vi "CV.vi"(2 "Run uninterrupted?":bool, 3 "Device Category IN:":string(combo)="ATLAS18SS" caption="Device Category:", 4 "Batch No.:":string, 5 "Sensor Serial No.:":string, 6 "DB Serial No.:":string) -> (0 "Done!":bool)   [LabVIEW 2019]
doc: "Performs CV measurements according to ATLAS ITk Quality Control Specifications."
uses:
  general_VIs/globals/QC_MeasurementSetup.vi
  general_VIs/globals/QC_RunInformation.vi
  InstrControl/InstrumentSetup.vi
  InstrControl/Switching/Switching.lvclass
  InstrControl/SupplyControl/SupplyControl.lvclass
  InstrControl/LCRControl/LCRControl.lvclass
  InstrControl/ArduinoControl/ArduinoControl.lvclass
  <vilib>/Analysis/NI_AALBase.lvlib
  InstrControl/InstrControl.lvclass
panel:
  out "Tab Control 2":enum32{"CV Setup", "CV Scan"}(tab)
  in  "V_depletion limit [V]":dbl=-300.0
  in  "step interval [s] IN":i32=5 caption="step interval [s]"
  in  "step [V] IN":dbl=10.0 caption="step [V]" format="%.1f"
  in  "Final volts [V] IN":dbl=-500.0 caption="Final volts [V]"
  in  "Initial volts [V] IN":dbl caption="Initial volts [V]"
  in  "Current Limit [µA]":dbl=1000.0 min=0.0001 format="%.3f"
  in  "Continue":bool
  in  "Quit":bool
  in  "Software current limit?":bool
  in  "Frequency [Hz] Setup":i32=500 caption="Frequency [Hz]" format="%#.3p"
  in  "Measurement Configurations":bool
  out "RH":dbl[](array[numeric]) caption="RH [%]" format="%#.2f"
  out "step interval [s]":u32=5
  out "step [V]":dbl=10.0 format="%.1f"
  out "Final volts [V]":dbl=-700.0 format="%.1f"
  out "Initial volts [V]":dbl format="%.1f"
  out "Frequency [Hz]":i32=1000 format="%#.3p"
  out "Temp.":dbl[](array[numeric]) caption="Temp. [°C]" format="%#.2f"
  out "Volts":dbl[](array[numeric]) caption="Volts [V]"
  out "Resistance":dbl[](array[numeric]) caption="Res [kOhm]"
  out "Capacitance":dbl[](array[numeric]) caption="Cap [pF]"
  out "Cgraph":cluster{"Initial volts":dbl, dbl, dbl[]}(graph)
  in  "Scales":T1(ring)
  in  "Cscale":enum16{"1/C^2 [1/nF^2]", "nF", "pF"}(ring)
  out "positive ramp?":bool
  out "Tab Control":enum32{"CV Setup", "CV Scan"}(tab)
  in  "Switching":string(combo)="Pickering Matrix"
  in  "LCR Meter":string(combo)="WayneKerr 6440B"
  in  "User:":string(combo)="Christoph"
  in  "CV Supply":string(combo)="Keithley 2410"
  in  "Hardware Configurations":bool
  in  "Temperature":enum16{"Read Arduino", "Enter manually"}(ring)
  in  "Manufacturer:":string(combo)="Hamamatsu"
  in  "abort":bool
  out "Device Category:":string
  out "DB Serial No.:":string
  out "Current Volts:":dbl format="%.2f"
  in  "quit (no save)":bool
  in  "Quit & Save":bool
  out "Bias On/Off:":bool
  out "STATUS 1":string
  out "Initiated:":string
  out "Sensor No.:":string
  out "No of steps":u32
  out "Current reading No.":u32
  out "Last reading at:":string
  # "Strip Sensor QC: CV"
  # "University of\nCambridge"
  # "Vertical Scale:"
  # "Measurement Configuration"
  # "CV Scan parameters:"
  # "Last 5 readings:"
  # "n-4"
  # "n-3"
  # "n-2"
  # "n-1"
  # "n"
  # "DUT Description"
  # "Hardware"
  # "DUT & Test Description:"
  # "Current status:"
  # "Rdg No:"
  # "out of"
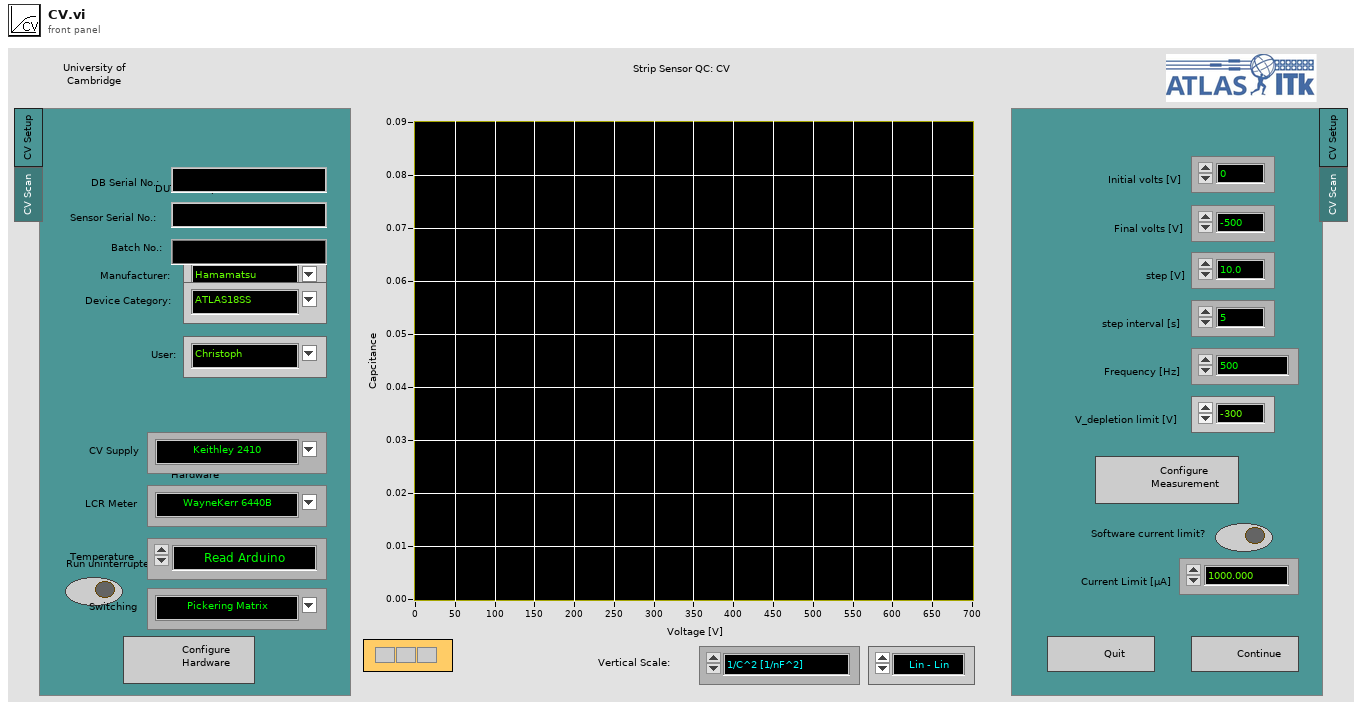
[diagram p1: front panel]
types:
  T1 = enum16{"Lin - Lin", "Log - Lin", "Lin - Log", "Log - log"}
  T2 = enum16{"Supply", "LCR", "Multimeter", "Switching"}
  T3 = enum16{"Reset", "Read Array", "Read Element", "Write Element", "Write Array", "Add Element", "Add Array"}
  T4 = enum16{"Reset", "Ground", "Striptest Bias", "Striptest SMU", "Striptest LCR", "IV", "CV", "Interstrip Cap", "Interstrip Res"}
  T5 = enum32{"IV", "CV", "Stability", "Striptest", "Cis", "Ris", "PTP"}
  T6 = cluster{"Sensor Serial No.:":string, "Wafer Serial No.:":string, "Batch:":string, "Manufacturer:":string, "Device Category:":string, "Database Serial No.:":string, "Date Initiated:":string, "Time Initiated:":string, "Test":string, "Instruments used:":string, "Probeplan used:":string, "End of Run comment:":string, "User:":string}
  T7 = cluster{"Institute":string, "Manufacturers":string[], "Devices":string[], "Serialnumbers Lookup DB":string, "Data directory":string, "Backup & screenshot directory":string, "List of known users":string[], "Measurement switch not used":bool, "Measurement Switch":string, "DUT Switch":string}
  T8 = cluster{"Supply":refnum<class "SupplyControl.lvclass">, "LCR":refnum<class "LCRControl.lvclass">, "Initial Voltage [V]":dbl, "Final Voltage [V]":dbl, "Step Size [V]":dbl, "Step Interval [s]":i32, "Number Of Steps":u32, "AC frequency [Hz]":i32, "RC Configuration":u16, "AC amplitude [V]":dbl, "Ramp down steps [V]":dbl, "Ramp down Interval [s]":i32, "Set Current Limit?":bool, "Current Limit [µA]":dbl, "Temperature Readout":enum16{"Read Arduino", "Enter manually"}, "Arduino":refnum<class "ArduinoControl.lvclass">, "Supply Name":string, "LCR Name":string, "V_depletion Limit [V]":dbl, "Switching":refnum<class "Switching.lvclass">, "Matrix used?":bool, "Matrix X Channels":cluster{"Bias Supply / SMU LO":i32, "Bias Supply / SMU HI":i32, "CV Box LO":i32, "CV Box HI":i32, "CV Box LO IN":i32, "CV Box HI IN":i32, "Volt meter LO":i32, "Volt meter HI":i32, "Mux1 C1":i32, "Mux1 C2":i32, "Mux2 C1":i32, "Mux2 C2":i32}}
  T9 = cluster{"VISA address":refnum<visa-resource-name>, "T sensor":enum16{"SHT", "DS"}, "Arduino":refnum<class "ArduinoControl.lvclass">}
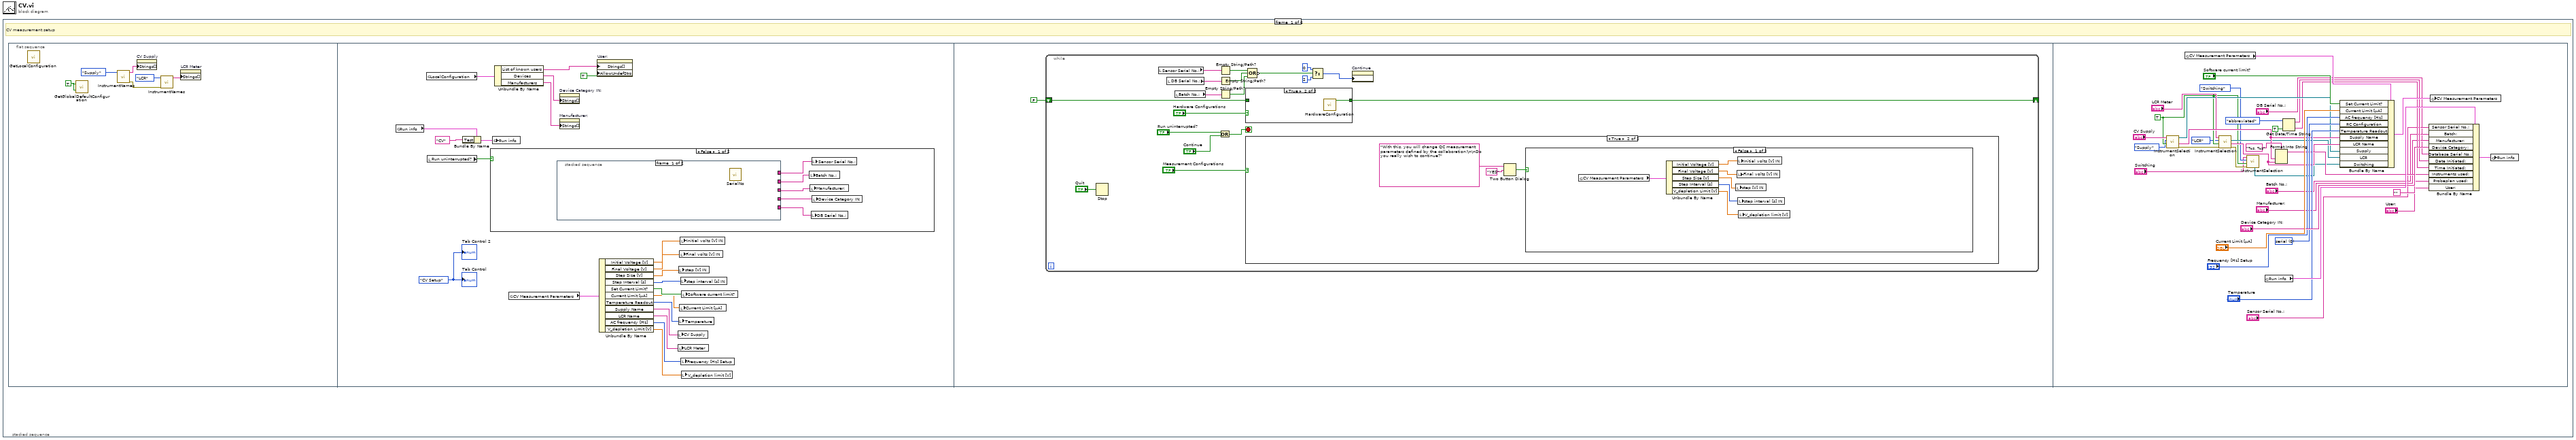
[diagram p0: block diagram]
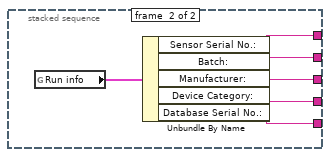
[diagram p2: hidden frame]
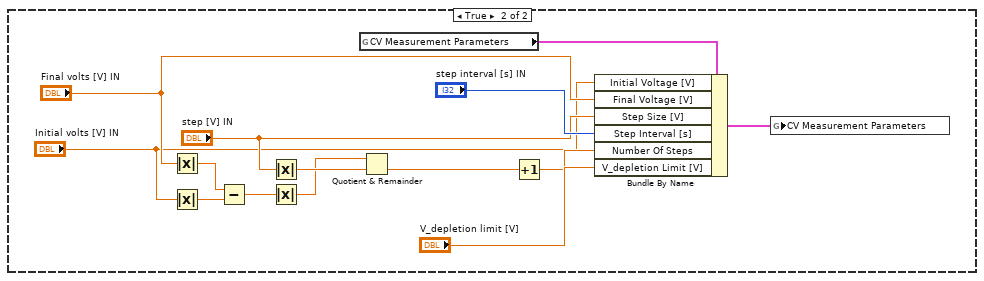
[diagram p6: hidden frame]
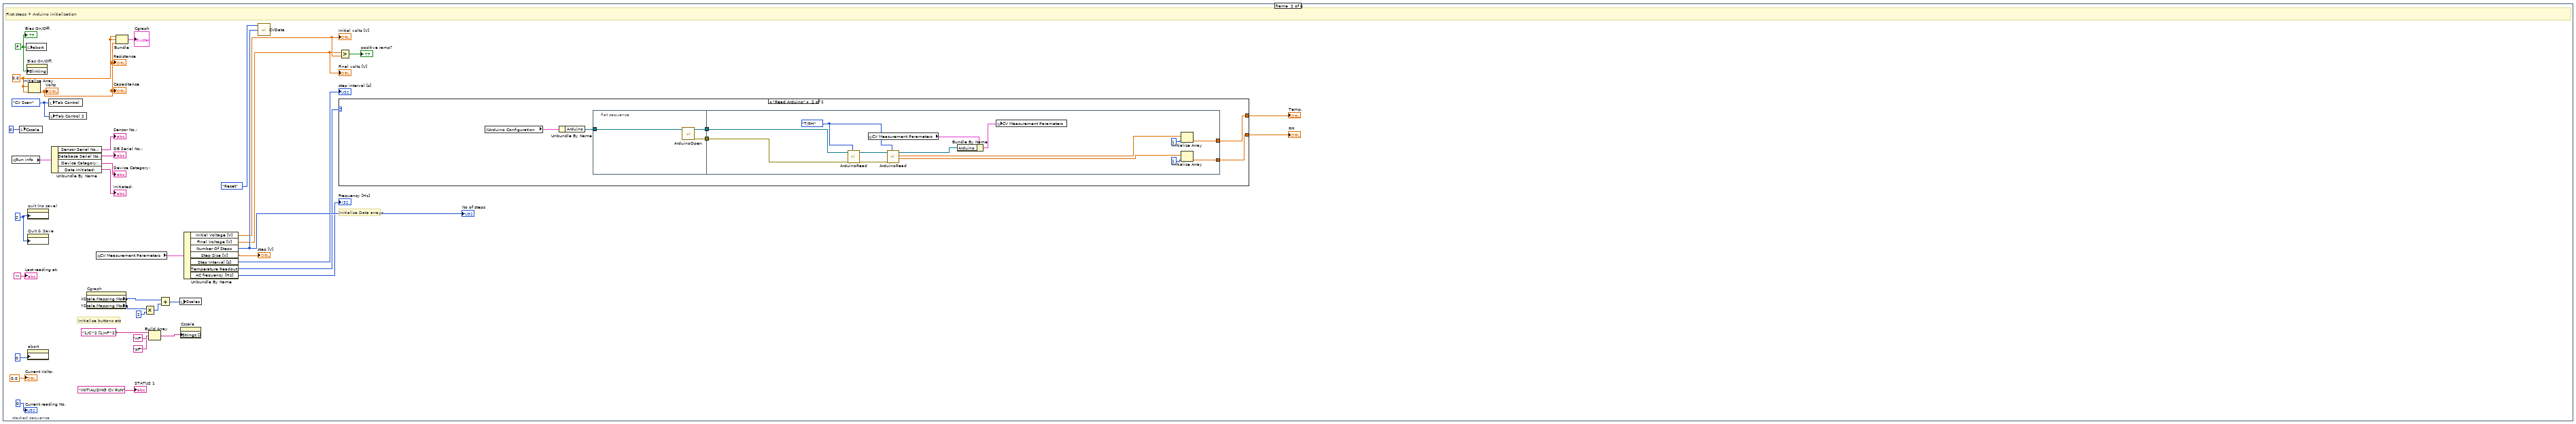
[diagram p7: hidden frame]
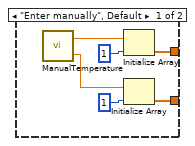
[diagram p8: hidden frame]
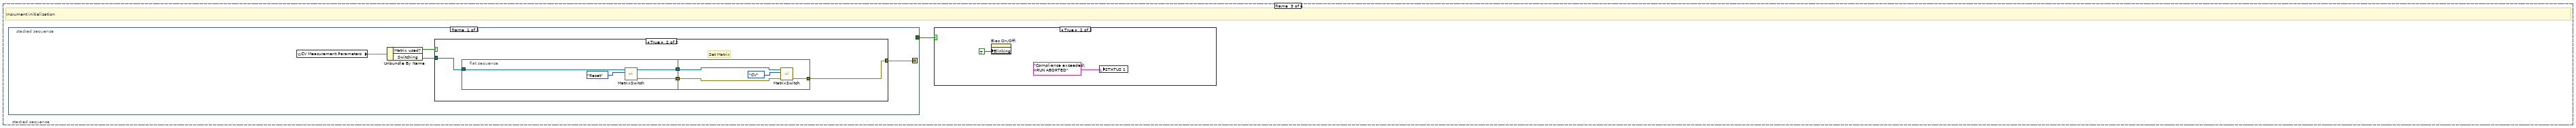
[diagram p9: hidden frame]
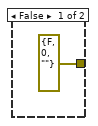
[diagram p10: hidden frame]
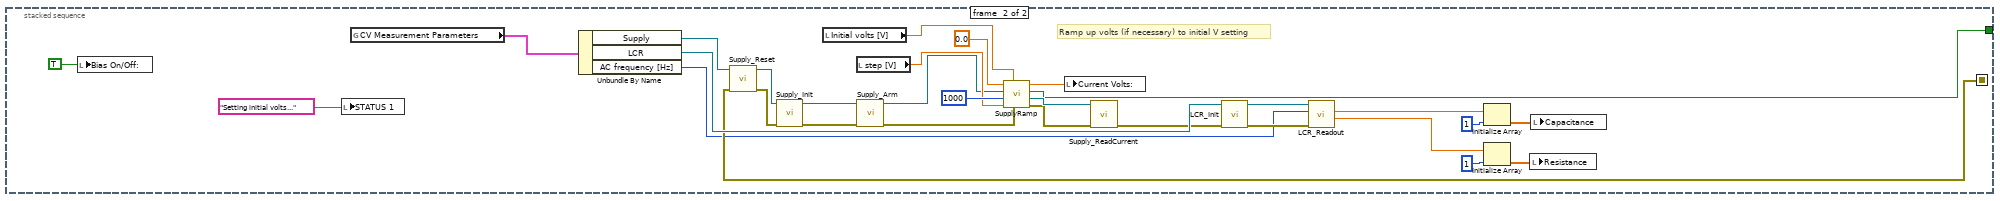
[diagram p11: hidden frame]
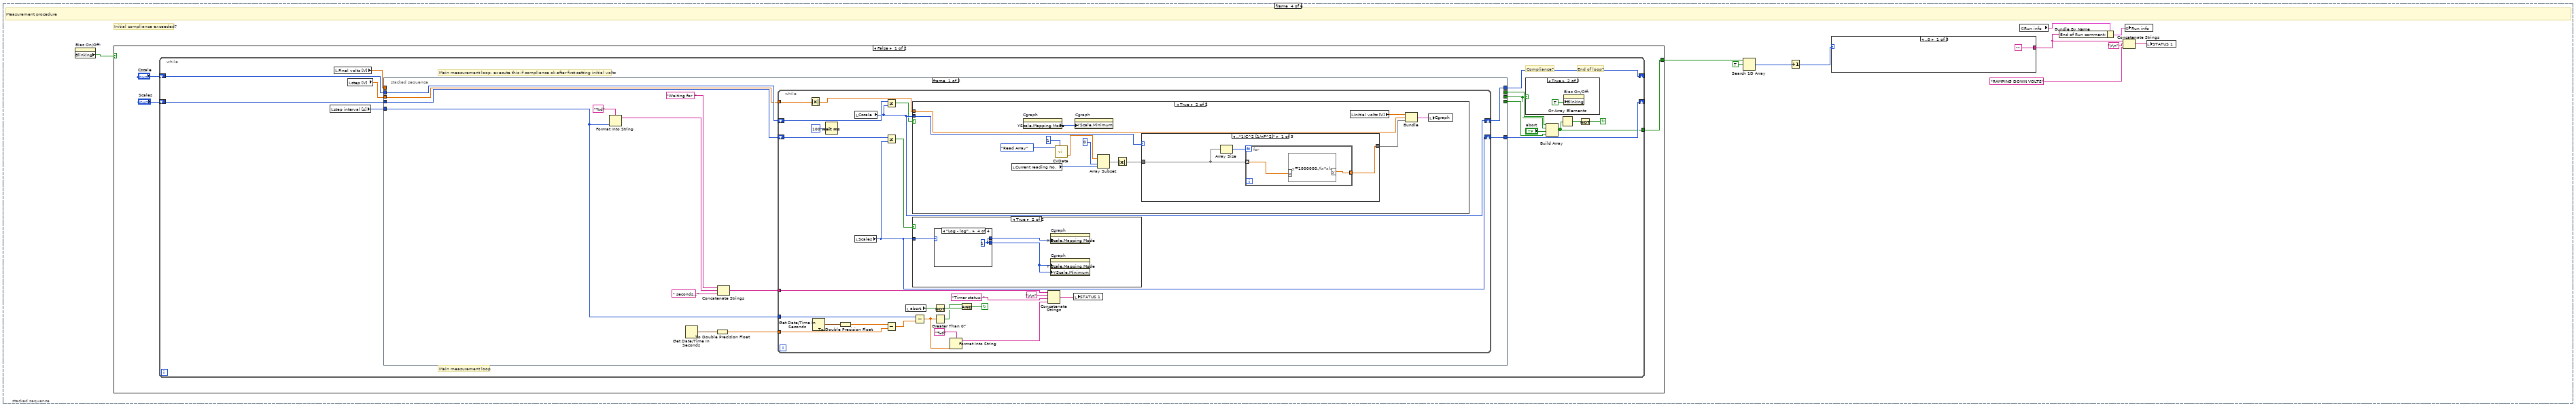
[diagram p13: hidden frame]
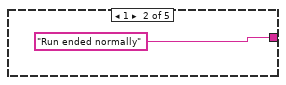
[diagram p14: hidden frame]
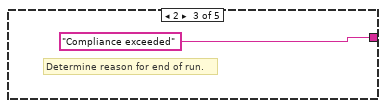
[diagram p15: hidden frame]
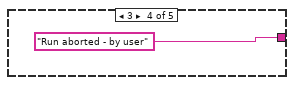
[diagram p16: hidden frame]
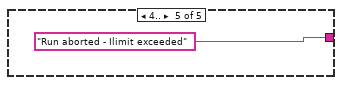
[diagram p17: hidden frame]
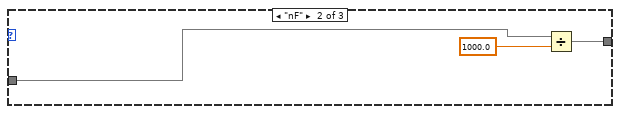
[diagram p19: hidden frame]
diagram:
  n1 = stacked-sequence {
    frame #0 {
      # "CV measurement setup"
      n2 = flat-sequence {
        frame #0 {
          w6 = TRUE
          n3 = call "GetLocalConfiguration.vi"() -> ()  [unwired: 3 in, 1 out]
          n4 = call "GetGlobalDefaultConfiguration.vi"("DO NOT override instruments"=w6, "Read defaults?"=w6) -> ()  [unwired: 1 in, 1 out]
          n5 = call "InstrumentNames.vi"("Instrument type"=T2."Supply") -> ("error out"=w1:errorcluster, "Instrument names"=w3:string[])  [unwired: 9 in]
          n6 = property on="CV Supply" class="CmbBox"("Strings[]"=w3) -> ()  [unwired: 2 in, 2 out]
          n7 = call "InstrumentNames.vi"("error in (no error)"=w1, "Instrument type"=T2."LCR") -> ("Instrument names"=w2:string[])  [unwired: 8 in, 1 out]
          n8 = property on="LCR Meter" class="CmbBox"("Strings[]"=w2) -> ()  [unwired: 2 in, 2 out]
        }
        frame #1 {
          w14 = enum32{"CV Setup", "CV Scan"}."CV Setup" ("Tab Control")
          n9 = global read "QC_RunInformation.vi" "Run info"() -> (w15:T6)
          n10 = global read "QC_RunInformation.vi" "LocalConfiguration"() -> (w23:T7)
          n11 = local read "Run uninterrupted?"() -> (w16:bool)
          n12 = Bundle By Name(cluster=w15, "Test"="CV") -> (w18:T6)
          n13 = case shown="False" w16 {
            frame False {
              n14 = stacked-sequence {
                tunnel: [_ w39] -> w32
                tunnel: [_ w38] -> w31
                tunnel: [_ w37] -> w30
                tunnel: [_ w36] -> w33
                tunnel: [_ w34] -> w29
                frame #0 {
                  n15 = call "SerialNo.vi"() -> ()  [unwired: 5 in, 1 out]
                }
                frame #1 {
                  n16 = global read "QC_RunInformation.vi" "Run info"() -> (w35:T6)
                  n17 = Unbundle By Name(w35) -> ("Sensor Serial No.:"=w39:string, "Batch:"=w38:string, "Manufacturer:"=w37:string, "Device Category:"=w36:string, "Database Serial No.:"=w34:string)
                }
              }
              n18 = local write "Batch No.:"(w31) -> ()
              n19 = local write "Manufacturer:"(w30) -> ()
              n20 = local write "DB Serial No.:"(w29) -> ()
              n21 = local write "Sensor Serial No.:"(w32) -> ()
              n22 = local write "Device Category IN:"(w33) -> ()
            }
            frame True {
            }
          }
          n23 = global write "QC_RunInformation.vi" "Run info"(w18) -> ()
          n24 = Unbundle By Name(w23) -> ("List of known users"=w22:string[], "Devices"=w7:string[], "Manufacturers"=w8:string[])
          n25 = global read "QC_MeasurementSetup.vi" "CV Measurement Parameters"() -> (w26:T8)
          n26 = property on="Device Category IN:" class="CmbBox"("Strings[]"=w7) -> ()  [unwired: 2 in, 2 out]
          n27 = property on="Manufacturer:" class="CmbBox"("Strings[]"=w8) -> ()  [unwired: 2 in, 2 out]
          n28 = property on="User:" class="CmbBox"("Strings[]"=w22, "AllowUndefStrs"=TRUE) -> ()  [unwired: 2 in, 2 out]
          n29 = Unbundle By Name(w26) -> ("Initial Voltage [V]"=w10:dbl, "Final Voltage [V]"=w11:dbl, "Step Size [V]"=w12:dbl, "Step Interval [s]"=w13:i32, "Set Current Limit?"=w25:bool, "Current Limit [µA]"=w24:dbl, "Temperature Readout"=w28:enum16{"Read Arduino", "Enter manually"}, "Supply Name"=w27:string, "LCR Name"=w20:string, "AC frequency [Hz]"=w19:i32, "V_depletion Limit [V]"=w9:dbl)
          n30 = local write "CV Supply"(w27) -> ()
          n31 = local write "LCR Meter"(w20) -> ()
          n32 = local write "step [V] IN"(w12) -> ()
          n33 = local write "Temperature"(w28) -> ()
          n34 = local write "Final volts [V] IN"(w11) -> ()
          n35 = local write "Current Limit [µA]"(w24) -> ()
          n36 = local write "Initial volts [V] IN"(w10) -> ()
          n37 = local write "step interval [s] IN"(w13) -> ()
          n38 = local write "Frequency [Hz] Setup"(w19) -> ()
          n39 = local write "V_depletion limit [V]"(w9) -> ()
          n40 = local write "Software current limit?"(w25) -> ()
          "Tab Control" <- w14
          "Tab Control 2" <- w14
        }
        frame #2 {
          n41 = while {
            shift-right: [w41] -> _
            shift-left: FALSE -> [w43]
            stop <- w45 stop-if-true
            n42 = Stop(stop? (T)="Quit") -> ()
            n43 = local read "Sensor Serial No.:"() -> (w57:string)
            n44 = local read "DB Serial No.:"() -> (w56:string)
            n45 = local read "Batch No.:"() -> (w49:string)
            n46 = Or(x="Run uninterrupted?", y="Continue") -> (x .or. y?=w45:bool)
            n47 = Empty String/Path?(string/path=w57) -> (empty?=w54:bool)
            n48 = Empty String/Path?(string/path=w56) -> (empty?=w55:bool)
            n49 = Empty String/Path?(string/path=w49) -> (empty?=w48:bool)
            n50 = case shown="True" "Hardware Configurations" {
              tunnel: [w59 w60] -> w41
              tunnel: w43 -> [w59 _]
              frame False {
              }
              frame True {
                n51 = call "HardwareConfiguration.vi"() -> ("configured?"=w60:bool)  [unwired: 11 in]
              }
            }
            n52 = case shown="True" "Measurement Configurations" {
              frame False {
              }
              frame True {
                n53 = Two Button Dialog(message="With this, you will change QC measurement parameters defined by the collaboration!\n\nDo you really wish to continue?", 2:"YES") -> (T button?=w61:bool)  [unwired: 1 in]
                n54 = case shown="False" w61 {
                  frame False {
                    n55 = global read "QC_MeasurementSetup.vi" "CV Measurement Parameters"() -> (w69:T8)
                    n56 = Unbundle By Name(w69) -> ("Initial Voltage [V]"=w66:dbl, "Final Voltage [V]"=w65:dbl, "Step Size [V]"=w67:dbl, "Step Interval [s]"=w68:i32, "V_depletion Limit [V]"=w64:dbl)
                    n57 = local write "step [V] IN"(w67) -> ()
                    n58 = local write "Final volts [V] IN"(w65) -> ()
                    n59 = local write "Initial volts [V] IN"(w66) -> ()
                    n60 = local write "step interval [s] IN"(w68) -> ()
                    n61 = local write "V_depletion limit [V]"(w64) -> ()
                  }
                  frame True {
                    n62 = Absolute Value(x="Final volts [V] IN") -> (abs(x)=w75:dbl)
                    n63 = Absolute Value(x="Initial volts [V] IN") -> (abs(x)=w76:dbl)
                    n64 = Subtract(x=w75, y=w76) -> (x-y=w79:dbl)
                    n65 = Absolute Value(x="step [V] IN") -> (abs(x)=w78:dbl)
                    n66 = Absolute Value(x=w79) -> (abs(x)=w77:dbl)
                    n67 = global read "QC_MeasurementSetup.vi" "CV Measurement Parameters"() -> (w83:T8)
                    n68 = Quotient & Remainder(x=w77, y=w78) -> (floor(x/y)=w74:dbl)  [unwired: 1 out]
                    n69 = Increment(x=w74) -> (x+1=w73:dbl)
                    n70 = Bundle By Name(cluster=w83, "Initial Voltage [V]"="Initial volts [V] IN", "Final Voltage [V]"="Final volts [V] IN", "Step Size [V]"="step [V] IN", "Step Interval [s]"="step interval [s] IN", "Number Of Steps"=w73, "V_depletion Limit [V]"="V_depletion limit [V]") -> (w82:T8)
                    n71 = global write "QC_MeasurementSetup.vi" "CV Measurement Parameters"(w82) -> ()
                  }
                }
              }
            }
            n72 = Compound Arithmetic op=OR(w54, w55, w48) -> (invert w53:bool)
            n73 = Select(t=0, s=w53, f=2) -> (s? t:f=w50:i32)
            n74 = property on="Continue" class="Bool"("DisabledEnum"=w50) -> ()  [unwired: 2 in, 2 out]
          }
        }
        frame #3 {
          w93 = TRUE
          w107 = u16 0 items=["serial", "parallel"] ("RC Configuration")
          n75 = call "InstrumentSelection.vi"("Verify GPIB address"=w93, "Instrument type"=T2."Supply", "Instrument name IN"="CV Supply") -> ("error out"=w99:errorcluster, "Instrument name OUT"=w102:string, "Supply"=w98:refnum<class "SupplyControl.lvclass">)  [unwired: 3 in, 3 out]
          n76 = global read "QC_MeasurementSetup.vi" "CV Measurement Parameters"() -> (w118:T8)
          n77 = call "InstrumentSelection.vi"("error in (no error)"=w99, "Verify GPIB address"=w93, "Instrument type"=T2."LCR", "Instrument name IN"="LCR Meter") -> ("error out"=w95:errorcluster, "Instrument name OUT"=w101:string, "LCR"=w97:refnum<class "LCRControl.lvclass">)  [unwired: 2 in, 3 out]
          n78 = call "InstrumentSelection.vi"("error in (no error)"=w95, "Verify GPIB address"=w93, "Instrument type"=T2."Switching", "Instrument name IN"="Switching") -> ("Switching"=w94:refnum<class "Switching.lvclass">)  [unwired: 2 in, 5 out]
          n79 = global read "QC_RunInformation.vi" "Run info"() -> (w113:T6)
          n80 = Format Into String(format string="%s, %s", w102, w101) -> (resulting string=w104:string)  [unwired: 2 in, 1 out]
          n81 = Get Date/Time String(date format (0)=enum16{"short", "long", "abbreviated"}."abbreviated", want seconds? (F)=TRUE) -> (date string=w90:string, time string=w89:string)  [unwired: 1 in]
          n82 = Bundle By Name(cluster=w118, "Set Current Limit?"="Software current limit?", "Current Limit [µA]"="Current Limit [µA]", "AC frequency [Hz]"="Frequency [Hz] Setup", "RC Configuration"=w107, "Temperature Readout"="Temperature", "Supply Name"=w102, "LCR Name"=w101, "Supply"=w98, "LCR"=w97, "Switching"=w94) -> (w119:T8)
          n83 = Bundle By Name(cluster=w113, "Sensor Serial No.:"="Sensor Serial No.:", "Batch:"="Batch No.:", "Manufacturer:"="Manufacturer:", "Device Category:"="Device Category IN:", "Database Serial No.:"="DB Serial No.:", "Date Initiated:"=w90, "Time Initiated:"=w89, "Instruments used:"=w104, "Probeplan used:"="", "User:"="User:") -> (w112:T6)
          n84 = global write "QC_MeasurementSetup.vi" "CV Measurement Parameters"(w119) -> ()
          n85 = global write "QC_RunInformation.vi" "Run info"(w112) -> ()
        }
      }
    }
    frame #1 {
      w121 = enum32{"CV Setup", "CV Scan"}."CV Scan" ("Tab Control")
      w139 = 2
      w146 = 0.0
      w138 = FALSE ("Visible")
      # "Initialise buttons etc"
      # "Initialise Data arrays"
      # "First steps + Arduino initialisation"
      n86 = global read "QC_RunInformation.vi" "Run info"() -> (w156:T6)
      n87 = local write "Cscale"(u16 0 ("Scale")) -> ()
      n88 = local write "abort"(w138) -> ()
      n89 = property on="Bias On/Off:" class="Bool (strict)"("Blinking"=w138) -> ()  [unwired: 2 in, 2 out]
      n90 = property on="quit (no save)" class="Bool"("DisabledEnum"=w139) -> ()  [unwired: 2 in, 2 out]
      n91 = property on="Quit & Save" class="Bool"("DisabledEnum"=w139) -> ()  [unwired: 2 in, 2 out]
      n92 = property on="abort" class="Bool (strict)"("DisabledEnum"=0) -> ()  [unwired: 2 in, 2 out]
      n93 = Initialize Array(w146, w146) -> (w123:dbl[])
      "Volts" <- w123
      "Capacitance" <- w123
      "Resistance" <- w123
      n94 = local write "Tab Control"(w121) -> ()
      n95 = local write "Tab Control 2"(w121) -> ()
      n96 = Unbundle By Name(w156) -> ("Sensor Serial No.:"=→"Sensor No.:":string, "Database Serial No.:"=→"DB Serial No.:":string, "Device Category:"=→"Device Category:":string, "Date Initiated:"=→"Initiated:":string)
      n97 = property on="Cgraph" class="WFGraph (strict)"() -> ("XScale.Mapping Mode"=w131:u8, "YScale.Mapping Mode"=w130:u8)  [unwired: 2 in, 2 out]
      n98 = global read "QC_MeasurementSetup.vi" "CV Measurement Parameters"() -> (w127:T8)
      n99 = Bundle(w146, w146, w123) -> (→"Cgraph":cluster{dbl, dbl, dbl[]})  [unwired: 1 in]
      n100 = Multiply(x=w130, y=2) -> (x*y=w133:i32)
      n101 = Build Array("1/C^2 [1/nF^2]", "nF", "pF") -> (w153:string[])
      n102 = Add(x=w131, y=w133) -> (x+y=w129:i32)
      n103 = local write "Scales"(w129) -> ()
      n104 = property on="Cscale" class="Enum (strict)"("Strings []"=w153) -> ()  [unwired: 2 in, 2 out]
      n105 = Unbundle By Name(w127) -> ("Initial Voltage [V]"=w137:dbl, "Final Voltage [V]"=w136:dbl, "Number Of Steps"=w147:u32, "Step Size [V]"=→"step [V]":dbl, "Step Interval [s]"=→"step interval [s]":i32, "Temperature Readout"=w140:enum16{"Read Arduino", "Enter manually"}, "AC frequency [Hz]"=→"Frequency [Hz]":i32)
      "No of steps" <- w147
      "Initial volts [V]" <- w137
      "Final volts [V]" <- w136
      n106 = call "CVData.vi"("Action"=T3."Reset", "Array Size / Index"=w147) -> ()  [unwired: 3 in, 2 out]
      n107 = case shown="\"Read Arduino\"" w140 {
        tunnel: [w162 w169] -> w143
        tunnel: [w159 w168] -> w128
        frame "Enter manually", Default {
          n108 = call "ManualTemperature.vi"() -> ("Humidity [%] out"=w158:dbl, "Temperature [°C] out"=w163:dbl)
          n109 = Initialize Array(w163, 1) -> (w162:dbl[])
          n110 = Initialize Array(w158, 1) -> (w159:dbl[])
        }
        frame "Read Arduino" {
          n111 = global read "InstrumentSetup.vi" "Arduino Configuration"() -> (w165:T9)
          n112 = Unbundle By Name(w165) -> ("Arduino"=w164:refnum<class "ArduinoControl.lvclass">)
          n113 = flat-sequence {
            tunnel: [w170] -> w167
            tunnel: [w172] -> w166
            tunnel: w164 -> [w171]
            tunnel: [w186] -> w169
            tunnel: [w183] -> w168
            tunnel: w167 -> [w175]
            tunnel: w166 -> [w176]
            frame #0 {
              n114 = call "ArduinoOpen.vi"("ArduinoControl in"=w171) -> ("error out"=w172:errorcluster, "ArduinoControl out"=w170:refnum<class "ArduinoControl.lvclass">)  [unwired: 9 in]
            }
            frame #1 {
              w177 = enum16{"T/RH", "Interlock", "Edgesense"}."T/RH" ("Arduino function")
              n115 = call "ArduinoRead.vi"("Arduino function"=w177, "error in (no error)"=w176, "ArduinoControl in"=w175) -> ("error out"=w173:errorcluster, "ArduinoControl out"=w174:refnum<class "ArduinoControl.lvclass">)  [unwired: 3 in, 4 out]
              n116 = global read "QC_MeasurementSetup.vi" "CV Measurement Parameters"() -> (w179:T8)
              n117 = call "ArduinoRead.vi"("Arduino function"=w177, "error in (no error)"=w173, "ArduinoControl in"=w174) -> ("rel. Humidity [%]"=w181:dbl, "Temperature [°C]"=w182:dbl, "ArduinoControl out"=w180:refnum<class "ArduinoControl.lvclass">)  [unwired: 3 in, 3 out]
              n118 = Bundle By Name(cluster=w179, "Arduino"=w180) -> (w178:T8)
              n119 = global write "QC_MeasurementSetup.vi" "CV Measurement Parameters"(w178) -> ()
              n120 = Initialize Array(w182, 1) -> (w186:dbl[])
              n121 = Initialize Array(w181, 1) -> (w183:dbl[])
            }
          }
        }
      }
      "Temp." <- w143
      "RH" <- w128
      n122 = Greater?(x=w136, y=w137) -> (0:→"positive ramp?":bool)
      "STATUS 1" <- "INITIALISING CV RUN"
      "Bias On/Off:" <- w138
      "Last reading at:" <- ""
      "Current reading No." <- u32 0 ("Current reading No.")
      "Current Volts:" <- 0.0 ("Current Volts:")
    }
    frame #2 {
      # "Insrument initialisation"
      n123 = stacked-sequence {
        seq-local: [w189 _] -> [_ w212]
        tunnel: [_ w216] -> w187
        frame #0 {
          n124 = global read "QC_MeasurementSetup.vi" "CV Measurement Parameters"() -> (w188:T8)
          n125 = Unbundle By Name(w188) -> ("Matrix used?"=w191:bool, "Switching"=w190:refnum<class "Switching.lvclass">)
          n126 = case shown="True" w191 {
            tunnel: w190 -> [_ w193]
            tunnel: [errorcluster {"status"=FALSE, "code"=0, "source"=""} ("error constant") w194] -> w189
            frame False {
            }
            frame True {
              # "Set Matrix"
              n127 = flat-sequence {
                tunnel: [w200] -> w196
                tunnel: [w199] -> w195
                tunnel: w193 -> [w198]
                tunnel: w196 -> [w204]
                tunnel: w195 -> [w203]
                tunnel: [w202] -> w194
                frame #0 {
                  n128 = call-dynamic "MatrixSwitch.vi"("Action"=T4."Reset", "Switching in"=w198) -> ("error out"=w200:errorcluster, "Switching out"=w199:refnum<class "Switching.lvclass">)  [unwired: 7 in, 1 out]
                }
                frame #1 {
                  n129 = call-dynamic "MatrixSwitch.vi"("error in (no error)"=w204, "Action"=T4."CV", "Switching in"=w203) -> ("error out"=w202:errorcluster)  [unwired: 6 in, 2 out]
                }
              }
            }
          }
        }
        frame #1 {
          # "Ramp up volts (if necessary) to initial V setting"
          n130 = local write "Bias On/Off:"(TRUE ("Compliance?")) -> ()
          n131 = local write "STATUS 1"("Setting initial volts..." ("STATUS 1")) -> ()
          n132 = global read "QC_MeasurementSetup.vi" "CV Measurement Parameters"() -> (w230:T8)
          n133 = Unbundle By Name(w230) -> ("Supply"=w227:refnum<class "SupplyControl.lvclass">, "LCR"=w226:refnum<class "LCRControl.lvclass">, "AC frequency [Hz]"=w205:i32)
          n134 = call-dynamic "Supply_Reset.vi"("error in (no error)"=w212, "SupplyControl in"=w227) -> ("error out"=w232:errorcluster, "SupplyControl out"=w234:refnum<class "SupplyControl.lvclass">)  [unwired: 8 in]
          n135 = call-dynamic "Supply_Init.vi"("error in (no error)"=w232, "SupplyControl in"=w234) -> ("error out"=w231:errorcluster, "SupplyControl out"=w233:refnum<class "SupplyControl.lvclass">)  [unwired: 8 in]
          n136 = local read "Initial volts [V]"() -> (w219:dbl)
          n137 = local read "step [V]"() -> (w220:dbl)
          n138 = call-dynamic "Supply_Arm.vi"("error in (no error)"=w231, "SupplyControl in"=w233) -> ("error out"=w214:errorcluster, "SupplyControl out"=w215:refnum<class "SupplyControl.lvclass">)  [unwired: 8 in]
          n139 = call "SupplyRamp.vi"("error in"=w214, "Requested Voltage"=w219, "Step Size"=w220, "Step Delay"=1000, "Supply IN"=w215, "Starting Voltage"=0.0) -> ("error out"=w217:errorcluster, "Supply OUT"=w218:refnum<class "SupplyControl.lvclass">, "Compliance exceeded"=w216:bool, "Current Voltage"=w223:dbl)  [unwired: 2 in]
          n140 = local write "Current Volts:"(w223) -> ()
          n141 = call-dynamic "Supply_ReadCurrent.vi"("error in (no error)"=w217, "SupplyControl in"=w218) -> ("error out"=w213:errorcluster)  [unwired: 7 in, 2 out]
          n142 = call-dynamic "LCR_Init.vi"("error in (no error)"=w213, "LCRControl in"=w226) -> ("error out"=w210:errorcluster, "LCRControl out"=w211:refnum<class "LCRControl.lvclass">)  [unwired: 8 in]
          n143 = call-dynamic "LCR_Readout.vi"("error in (no error)"=w210, "Frequency in Hz"=w205, "LCRControl in"=w211) -> ("Resistance in Ohm"=w207:dbl, "Capacitance in pF"=w209:dbl)  [unwired: 5 in, 2 out]
          n144 = Initialize Array(w209, 1) -> (w224:dbl[])
          n145 = Initialize Array(w207, 1) -> (w206:dbl[])
          n146 = local write "Resistance"(w206) -> ()
          n147 = local write "Capacitance"(w224) -> ()
        }
      }
      n148 = case shown="True" w187 {
        frame False {
        }
        frame True {
          n149 = property on="Bias On/Off:" class="Bool (strict)"("Blinking"=TRUE) -> ()  [unwired: 2 in, 2 out]
          n150 = local write "STATUS 1"("Compliance exceeded\nRUN ABORTED") -> ()
        }
      }
    }
    frame #3 {
      # "Initial compliance exceeded?"
      # "Measurement procedure"
      n151 = property on="Bias On/Off:" class="Bool (strict)"() -> ("Blinking"=w247:bool)  [unwired: 2 in, 2 out]
      n152 = case shown="False" w247 {
        tunnel: [w255 w502] -> w246
        frame False {
          n153 = while {
            shift-left: "Cscale" -> [w265]
            shift-right: [w264] -> _
            shift-left: "Scales" -> [w266]
            shift-right: [w267] -> _
            tunnel: [w263] -> w255
            stop <- w268 continue-if-true
            # "Main measurement loop"
            # "End of loop?"
            # "Compliance?"
            # "Main measurement loop. execute this if compliance ok after first setting initial volts"
            n154 = local read "step interval [s]"() -> (w260:u32)
            n155 = local read "Final volts [V]"() -> (w261:dbl)
            n156 = local read "step [V]"() -> (w262:dbl)
            n157 = stacked-sequence {
              tunnel: [w282 _] -> w267
              tunnel: w262 -> [w279 w345]
              tunnel: [_ w344] -> w257
              tunnel: w261 -> [_ w343]
              tunnel: w260 -> [w270 w342]
              tunnel: [_ w341] -> w259
              tunnel: w266 -> [w281 _]
              tunnel: w265 -> [w280 _]
              tunnel: [w278 _] -> w264
              tunnel: [_ w339] -> w258
              frame #0 {
                n158 = Format Into String(format string="%d", w270) -> (resulting string=w275:string)  [unwired: 2 in, 1 out]
                n159 = Get Date/Time In Seconds() -> (seconds since 1Jan1904=w272:timestamp)
                n160 = To Double Precision Float(number=w272) -> (double precision float=w273:dbl)
                n161 = Concatenate Strings("Waiting for  ", w275, " seconds...") -> (w271:string)
                n162 = while {
                  tunnel: w279 -> [w291]
                  shift-left: w280 -> [w295]
                  shift-right: [w288] -> w278
                  shift-left: w281 -> [w296]
                  shift-right: [w297] -> w282
                  tunnel: w271 -> [w289]
                  tunnel: w270 -> [w301]
                  tunnel: w273 -> [w302]
                  stop <- w303 continue-if-true
                  n163 = Absolute Value(x=w291) -> (abs(x)=w290:dbl)
                  n164 = Get Date/Time In Seconds() -> (seconds since 1Jan1904=w287:timestamp)
                  n165 = Wait (ms)(milliseconds to wait=u32 100) -> ()  [unwired: 1 out]
                  n166 = To Double Precision Float(number=w287) -> (double precision float=w307:dbl)
                  n167 = local read "Cscale"() -> (w288:enum16{"1/C^2 [1/nF^2]", "nF", "pF"})
                  n168 = local read "Scales"() -> (w297:T1)
                  n169 = Not Equal?(x=w295, y=w288) -> (x != y?=w286:bool)
                  n170 = Not Equal?(x=w296, y=w297) -> (x != y?=w298:bool)
                  n171 = Subtract(x=w307, y=w302) -> (x-y=w284:dbl)
                  n172 = local read "abort"() -> (w300:bool)
                  n173 = case shown="True" w286 {
                    tunnel: w290 -> [_ w319]
                    tunnel: w288 -> [_ w312]
                    frame False {
                    }
                    frame True {
                      n174 = local read "Current reading No."() -> (w317:u32)
                      n175 = property on="Cgraph" class="WFGraph (strict)"() -> ("YScale.Mapping Mode"=w314:u8)  [unwired: 2 in, 2 out]
                      n176 = call "CVData.vi"("Action"=T3."Read Array", "Array No."=u32 1 ("Action")) -> ("Array OUT"=w308:dbl[])  [unwired: 3 in, 1 out]
                      n177 = property on="Cgraph" class="WFGraph (strict)"("YScale.Minimum"=w314) -> ()  [unwired: 2 in, 2 out]
                      n178 = Array Subset(array=w308, index=0, length=w317) -> (w315:dbl[])
                      n179 = Absolute Value(x=w315) -> (abs(x)=w313:dbl[])
                      n180 = case shown="..\"1/C^2 [1/nF^2]\"" w312 {
                        tunnel: [w323 w326 w329] -> w311
                        tunnel: w313 -> [w321 w328 w329]
                        frame .."1/C^2 [1/nF^2]" {
                          n181 = Array Size(array=w321) -> (size(s)=w322:i32)
                          n182 = for {
                            N: w322 -> [_]
                            tunnel: w321 -> [w325] mode=indexing
                            tunnel: [w324] -> w323 mode=indexing
                            n183 = formula code="y=1000000./(x*x);"("x"=w325) -> ("y"=w324:dbl)
                          }
                        }
                        frame "nF" {
                          n184 = Divide(x=w328, y=1000.0) -> (x/y=w326:dbl[])
                        }
                        frame "pF".. {
                        }
                      }
                      n185 = local read "Initial volts [V]"() -> (w318:dbl)
                      n186 = Bundle("Initial volts [V]"=w318, w319, w311) -> (w316:cluster{"Initial volts [V]":dbl, dbl, dbl[]})  [unwired: 1 in]
                      n187 = local write "Cgraph"(w316) -> ()
                    }
                  }
                  n188 = case shown="True" w298 {
                    tunnel: w297 -> [_ w332]
                    frame False {
                    }
                    frame True {
                      n189 = case shown="\"Log - log\".." w332 {
                        tunnel: [w333 1 0 w338] -> w331
                        tunnel: [w333 0 1 w338] -> w330
                        frame .."Lin - Lin" {
                          w333 = 0
                        }
                        frame "Log - Lin" {
                        }
                        frame "Lin - Log" {
                        }
                        frame "Log - log".. {
                          w338 = 1
                        }
                      }
                      n190 = property on="Cgraph" class="WFGraph (strict)"("X Scale.Mapping Mode"=w331) -> ()  [unwired: 2 in, 2 out]
                      n191 = property on="Cgraph" class="WFGraph (strict)"("Y Scale.Mapping Mode"=w330, "YScale.Minimum"=w330) -> ()  [unwired: 2 in, 2 out]
                    }
                  }
                  n192 = Subtract(x=w301, y=w284) -> (x-y=w283:dbl)
                  n193 = Not(x=w300) -> (.not. x?=w306:bool)
                  n194 = Greater Than 0?(x=w283) -> (x > 0?=w285:bool)
                  n195 = Format Into String(format string="%d", w283) -> (resulting string=w305:string)  [unwired: 2 in, 1 out]
                  n196 = And(x=w285, y=w306) -> (x .and. y?=w303:bool)
                  n197 = Concatenate Strings(w289, "\r\n", "Timer status: ", w305) -> (w299:string)
                  n198 = local write "STATUS 1"(w299) -> ()
                }
              }
              frame #1 {
                n199 = local read "abort"() -> (w340:bool)
                n200 = case shown="False" w340 {
                  tunnel: [w351 w499] -> w341
                  tunnel: w342 -> [w350 _]
                  tunnel: w343 -> [w349 _]
                  tunnel: [w347 w499] -> w344
                  tunnel: w345 -> [w348 _]
                  tunnel: [w346 w499] -> w339
                  frame False {
                    n201 = stacked-sequence {
                      seq-local: [w377 _ _] -> [_ w401 _]
                      seq-local: [w376 _ _] -> [_ _ w468]
                      seq-local: [w363 _ _] -> [_ _ w469]
                      tunnel: w348 -> [_ w413 w474]
                      tunnel: w349 -> [_ _ w465]
                      tunnel: [_ _ w472] -> w351
                      tunnel: [_ _ w471] -> w347
                      tunnel: w350 -> [_ _ _]
                      tunnel: [w379 _ _] -> w346
                      frame #0 {
                        w359 = T3."Write Element" ("Action")
                        # "SMU data"
                        n202 = Get Date/Time String(want seconds? (F)=TRUE) -> (time string=w378:string)  [unwired: 2 in, 1 out]
                        n203 = local write "Last reading at:"(w378) -> ()
                        n204 = local write "STATUS 1"("Reading LCR meter..." ("status")) -> ()
                        n205 = global read "QC_MeasurementSetup.vi" "CV Measurement Parameters"() -> (w375:T8)
                        n206 = Unbundle By Name(w375) -> ("Temperature Readout"=w353:enum16{"Read Arduino", "Enter manually"}, "Arduino"=w352:refnum<class "ArduinoControl.lvclass">, "LCR"=w369:refnum<class "LCRControl.lvclass">, "AC frequency [Hz]"=w354:i32, "Supply"=w370:refnum<class "SupplyControl.lvclass">, "Set Current Limit?"=w374:bool, "Current Limit [µA]"=w372:dbl)
                        n207 = local read "Current reading No."() -> (w358:u32)
                        n208 = case shown="\"Read Arduino\"" w353 {
                          tunnel: [w386 w389] -> w356
                          tunnel: [w383 w392] -> w361
                          tunnel: w352 -> [_ w391]
                          frame "Enter manually", Default {
                            n209 = local read "Temp."() -> (w388:dbl[])
                            n210 = local read "RH"() -> (w384:dbl[])
                            n211 = Index Array(array=w388, index=0) -> (element=w386:dbl)
                            n212 = Index Array(array=w384, index=0) -> (element=w383:dbl)
                          }
                          frame "Read Arduino" {
                            n213 = call "ArduinoRead.vi"("Arduino function"=enum16{"T/RH", "Interlock", "Edgesense"}."T/RH", "ArduinoControl in"=w391) -> ("rel. Humidity [%]"=w392:dbl, "Temperature [°C]"=w389:dbl)  [unwired: 4 in, 4 out]
                          }
                        }
                        n214 = local read "Current Volts:"() -> (w362:dbl)
                        n215 = Multiply(x=w372, y=1000.0) -> (x*y=w371:dbl)
                        n216 = call-dynamic "Supply_ReadCurrent.vi"("SupplyControl in"=w370) -> ("error out"=w364:errorcluster, "Current in nA"=w380:dbl, "SupplyControl out"=w376:refnum<class "SupplyControl.lvclass">)  [unwired: 8 in]
                        n217 = case shown="True" w374 {
                          tunnel: w380 -> [_ w397]
                          tunnel: w371 -> [_ w395]
                          tunnel: [FALSE w394] -> w379
                          frame False {
                          }
                          frame True {
                            n218 = Absolute Value(x=w397) -> (abs(x)=w396:dbl)
                            n219 = Greater?(x=w396, y=w395) -> (0:w394:bool)
                          }
                        }
                        n220 = call "CVData.vi"("Action"=w359, "Array No."=0, "Array Size / Index"=w358, "Data IN"=w362) -> ()  [unwired: 1 in, 2 out]
                        n221 = call-dynamic "LCR_Readout.vi"("error in (no error)"=w364, "Frequency in Hz"=w354, "LCRControl in"=w369) -> ("error out"=w363:errorcluster, "Resistance in Ohm"=w357:dbl, "Capacitance in pF"=w355:dbl)  [unwired: 5 in, 1 out]
                        n222 = Increment(x=w358) -> (x+1=w377:u32)
                        n223 = local write "Current reading No."(w377) -> ()
                        n224 = call "CVData.vi"("Action"=w359, "Array No."=u32 1, "Array Size / Index"=w358, "Data IN"=w355) -> ()  [unwired: 1 in, 2 out]
                        n225 = call "CVData.vi"("Action"=w359, "Array No."=u32 2, "Array Size / Index"=w358, "Data IN"=w357) -> ()  [unwired: 1 in, 2 out]
                        n226 = call "CVData.vi"("Action"=w359, "Array No."=u32 3, "Array Size / Index"=w358, "Data IN"=w356) -> ()  [unwired: 1 in, 2 out]
                        n227 = call "CVData.vi"("Action"=w359, "Array No."=u32 4, "Array Size / Index"=w358, "Data IN"=w361) -> ()  [unwired: 1 in, 2 out]
                      }
                      frame #1 {
                        w410 = u32 5 ("y")
                        # "Update plots"
                        n228 = property on="Cgraph" class="WFGraph (strict)"() -> ("YScale.Mapping Mode"=w402:u8)  [unwired: 2 in, 2 out]
                        n229 = Greater?(x=w401, y=w410) -> (0:w409:bool)
                        n230 = call "CVData.vi"("Action"=T3."Read Array", "Array No."=1) -> ("Array OUT"=w399:dbl[])  [unwired: 3 in, 1 out]
                        n231 = case shown="True" w409 {
                          tunnel: w401 -> [w418 w421]
                          tunnel: w410 -> [_ w420]
                          tunnel: [w418 w420] -> w408
                          tunnel: [0 w419] -> w406
                          frame False {
                          }
                          frame True {
                            n232 = Subtract(x=w421, y=w420) -> (x-y=w419:u32)
                          }
                        }
                        n233 = property on="Cgraph" class="WFGraph (strict)"("YScale.Minimum"=w402) -> ()  [unwired: 2 in, 2 out]
                        n234 = Array Subset(array=w399, index=0, length=w401) -> (w405:dbl[])
                        n235 = local read "Cscale"() -> (w411:enum16{"1/C^2 [1/nF^2]", "nF", "pF"})
                        n236 = Absolute Value(x=w405) -> (abs(x)=w404:dbl[])
                        n237 = case shown="..\"1/C^2 [1/nF^2]\"" w411 {
                          tunnel: [w454 w457 w460] -> w416
                          tunnel: w404 -> [w452 w459 w460]
                          frame .."1/C^2 [1/nF^2]" {
                            n238 = Array Size(array=w452) -> (size(s)=w453:i32)
                            n239 = for {
                              N: w453 -> [_]
                              tunnel: w452 -> [w456] mode=indexing
                              tunnel: [w455] -> w454 mode=indexing
                              n240 = formula code="y=1000000./(x*x);"("x"=w456) -> ("y"=w455:dbl)
                            }
                          }
                          frame "nF" {
                            n241 = Divide(x=w459, y=1000.0) -> (x/y=w457:dbl[])
                          }
                          frame "pF".. {
                          }
                        }
                        n242 = for {
                          N: 5 -> [_]
                          tunnel: w408 -> [w427]
                          tunnel: w406 -> [w426]
                          tunnel: w401 -> [w425]
                          i -> [w423]
                          n243 = call "CVData.vi"("Action"=T3."Read Array", "Array No."=w423) -> ("Array OUT"=w422:dbl[])  [unwired: 3 in, 1 out]
                          n244 = case shown="2" w423 {
                            tunnel: w427 -> [w430 w434 w439 _ _]
                            tunnel: w426 -> [w431 w435 w440 _ _]
                            tunnel: w422 -> [w429 w433 w441 w445 w450]
                            tunnel: w425 -> [_ _ _ w443 w448]
                            frame ..0 {
                              n245 = Array Subset(array=w429, index=w431, length=w430) -> (w428:dbl[])
                              n246 = local write "Volts"(w428) -> ()
                            }
                            frame 1 {
                              n247 = Array Subset(array=w433, index=w435, length=w434) -> (w432:dbl[])
                              n248 = local write "Capacitance"(w432) -> ()
                            }
                            frame 2 {
                              n249 = Array Subset(array=w441, index=w440, length=w439) -> (w438:dbl[])
                              n250 = Multiply(x=w438, y=0.001) -> (x*y=w437:dbl[])
                              n251 = local write "Resistance"(w437) -> ()
                            }
                            frame 3 {
                              n252 = Decrement(x=w443) -> (x-1=w442:u32)
                              n253 = Array Subset(array=w445, index=w442, length=1) -> (w444:dbl[])
                              n254 = local write "Temp."(w444) -> ()
                            }
                            frame 4.. {
                              n255 = Decrement(x=w448) -> (x-1=w447:u32)
                              n256 = Array Subset(array=w450, index=w447, length=1) -> (w449:dbl[])
                              n257 = local write "RH"(w449) -> ()
                            }
                          }
                        }
                        n258 = local read "Initial volts [V]"() -> (w414:dbl)
                        n259 = Absolute Value(x=w413) -> (abs(x)=w412:dbl)
                        n260 = Bundle("Initial volts [V]"=w414, w412, w416) -> (w403:cluster{"Initial volts [V]":dbl, dbl, dbl[]})  [unwired: 1 in]
                        n261 = local write "Cgraph"(w403) -> ()
                      }
                      frame #2 {
                        # "Increment volts and check for end of loop"
                        n262 = local read "positive ramp?"() -> (w470:bool)
                        n263 = local read "Current Volts:"() -> (w466:dbl)
                        n264 = case shown="True" w470 {
                          tunnel: w465 -> [w477 w481]
                          tunnel: w474 -> [w478 w484]
                          tunnel: [w476 w483] -> w461
                          tunnel: [w475 w480] -> w473
                          tunnel: w466 -> [w479 w482]
                          frame False {
                            n265 = Subtract(x=w479, y=w478) -> (x-y=w475:dbl)
                            n266 = Greater Or Equal?(x=w475, y=w477) -> (x >= y?=w476:bool)
                          }
                          frame True {
                            n267 = Add(x=w482, y=w484) -> (x+y=w480:dbl)
                            n268 = Less Or Equal?(x=w480, y=w481) -> (x <= y?=w483:bool)
                          }
                        }
                        n269 = Quotient & Remainder(x=w466, y=w465) -> (x-y*floor(x/y)=w467:dbl, floor(x/y)=w464:dbl)
                        n270 = Not Equal To 0?(x=w467) -> (x != 0?=w462:bool)
                        n271 = Equal To 0?(x=w464) -> (x = 0?=w463:bool)
                        n272 = Or(x=w462, y=w463) -> ()  [unwired: 1 out]
                        n273 = case shown="True" w461 {
                          tunnel: w473 -> [_ w495]
                          tunnel: [TRUE FALSE] -> w472
                          tunnel: [FALSE w496] -> w471
                          tunnel: w466 -> [_ w493]
                          tunnel: w469 -> [_ w492]
                          tunnel: w468 -> [_ w491]
                          frame False {
                          }
                          frame True {
                            n274 = local read "step [V]"() -> (w489:dbl)
                            n275 = call "SupplyRamp.vi"("error in"=w492, "Requested Voltage"=w495, "Step Size"=w489, "Step Delay"=100, "Supply IN"=w491, "Starting Voltage"=w493) -> ("error out"=w487:errorcluster, "Compliance exceeded"=w496:bool, "Current Voltage"=w490:dbl)  [unwired: 2 in, 1 out]
                            n276 = case shown="No Error" w487 {
                              tunnel: w490 -> [w498 _]
                              frame No Error {
                                n277 = local write "Current Volts:"(w498) -> ()
                              }
                              frame Error {
                              }
                            }
                            n278 = property on="Bias On/Off:" class="Bool (strict)"("Blinking"=w496) -> ()  [unwired: 2 in, 2 out]
                            n279 = local write "STATUS 1"("Incrementing volts.") -> ()
                          }
                        }
                      }
                    }
                  }
                  frame True {
                    w499 = FALSE
                  }
                }
              }
            }
            n280 = case shown="True" w257 {
              frame False {
              }
              frame True {
                n281 = property on="Bias On/Off:" class="Bool (strict)"("Blinking"=TRUE) -> ()  [unwired: 2 in, 2 out]
              }
            }
            n282 = Build Array(w259, w257, "abort", w258) -> (w263:bool[])
            n283 = Or Array Elements(Boolean array=w263) -> (logical OR=w269:bool)
            n284 = Not(x=w269) -> (.not. x?=w268:bool)
          }
        }
        frame True {
          w501 = FALSE
          # "compliance was exceeded when first voltage applied."
          # "Flag compliance as reason for end of run"
          n285 = local write "STATUS 1"("Run aborted - compliance exceeded.") -> ()
          n286 = Build Array(w501, TRUE, w501, w501) -> (w502:bool[])
        }
      }
      n287 = Search 1D Array(1D array=w246, element=TRUE) -> (index of element=w244:i32)  [unwired: 1 in]
      n288 = Increment(x=w244) -> (x+1=w243:i32)
      n289 = case shown="..0" w243 {
        tunnel: ["" "Run ended normally" "Compliance exceeded" "Run aborted - by user" "Run aborted - Ilimit exceeded"] -> w238
        frame ..0 {
        }
        frame 1 {
        }
        frame 2 {
          # "Determine reason for end of run."
        }
        frame 3 {
        }
        frame 4.. {
        }
      }
      n290 = global read "QC_RunInformation.vi" "Run info"() -> (w242:T6)
      n291 = Bundle By Name(cluster=w242, "End of Run comment:"=w238) -> (w237:T6)
      n292 = Concatenate Strings(w238, "\r\n", "RAMPING DOWN VOLTS") -> (w241:string)
      n293 = global write "QC_RunInformation.vi" "Run info"(w237) -> ()
      n294 = local write "STATUS 1"(w241) -> ()
    }
    frame #4 {
      # "Ramp down and switch off supply"
      n295 = stacked-sequence {
        frame #0 {
          # "Tie up loose ends. Set volts to zero and switch to standby"
          # "Ramp down volts now"
          n296 = global read "QC_MeasurementSetup.vi" "CV Measurement Parameters"() -> (w513:T8)
          n297 = Unbundle By Name(w513) -> ("Supply"=w510:refnum<class "SupplyControl.lvclass">, "Ramp down steps [V]"=w512:dbl, "Ramp down Interval [s]"=w511:i32, "Switching"=w506:refnum<class "Switching.lvclass">, "Matrix used?"=w505:bool)
          n298 = local read "Current Volts:"() -> (w518:dbl)
          n299 = Multiply(x=w511, y=1000) -> (x*y=w515:i32)
          n300 = call "SupplyRamp.vi"("Requested Voltage"=0.0, "Step Size"=w512, "Step Delay"=w515, "Supply IN"=w510, "Starting Voltage"=w518) -> ("error out"=w508:errorcluster, "Supply OUT"=w509:refnum<class "SupplyControl.lvclass">, "Current Voltage"=w516:dbl)  [unwired: 3 in, 1 out]
          n301 = call-dynamic "Supply_Stby.vi"("error in (no error)"=w508, "SupplyControl in"=w509) -> ("error out"=w507:errorcluster)  [unwired: 8 in, 1 out]
          n302 = local write "Current Volts:"(w516) -> ()
          n303 = case shown="True" w505 {
            tunnel: w506 -> [_ w523]
            tunnel: w507 -> [_ w522]
            frame False {
            }
            frame True {
              n304 = call-dynamic "MatrixSwitch.vi"("error in (no error)"=w522, "Action"=T4."Reset", "Switching in"=w523) -> ("error out"=w519:errorcluster, "Switching out"=w520:refnum<class "Switching.lvclass">)  [unwired: 6 in, 1 out]
              n305 = call-dynamic "Close.vi"("error in (no error)"=w519, "Switching in"=w520) -> ()  [unwired: 8 in, 2 out]
            }
          }
        }
        frame #1 {
          w528 = 0
          n306 = local write "Bias On/Off:"(FALSE ("Visible")) -> ()
          n307 = local write "Current Volts:"(0.0 ("Current Volts:")) -> ()
          n308 = property on="abort" class="Bool (strict)"("DisabledEnum"=2) -> ()  [unwired: 2 in, 2 out]
          n309 = property on="Quit & Save" class="Bool"("DisabledEnum"=w528) -> ()  [unwired: 2 in, 2 out]
          n310 = property on="quit (no save)" class="Bool"("DisabledEnum"=w528) -> ()  [unwired: 2 in, 2 out]
          n311 = local write "STATUS 1"("Run finished. \nSave data?" ("STATUS 1")) -> ()
        }
        frame #2 {
          n312 = Current VI's Path() -> (path=w530:path)
          n313 = call "SaveJPEG.vi"("Test"="CV", "File Path Control"=w530) -> ()  [unwired: 1 in, 2 out]
        }
      }
    }
    frame #5 {
      # "Loop and await decision on whether to save or junk data"
      # "Display and save data"
      n314 = local read "Scales"() -> (w541:T1)
      n315 = local read "Cscale"() -> (w540:enum16{"1/C^2 [1/nF^2]", "nF", "pF"})
      n316 = while {
        shift-left: w540 -> [w591]
        shift-right: [w590] -> _
        shift-left: w541 -> [w593]
        shift-right: [w592] -> _
        tunnel: ["Quit & Save"] -> w543
        tunnel: ["quit (no save)"] -> w542
        stop <- w588 continue-if-true
        n317 = local read "Scales"() -> (w592:T1)
        n318 = local read "Cscale"() -> (w590:enum16{"1/C^2 [1/nF^2]", "nF", "pF"})
        n319 = Not Equal?(x=w593, y=w592) -> (x != y?=w586:bool)
        n320 = Not Equal?(x=w591, y=w590) -> (x != y?=w585:bool)
        n321 = case shown="True" w586 {
          tunnel: w592 -> [_ w620]
          frame False {
          }
          frame True {
            n322 = case shown="..\"Lin - Lin\"" w620 {
              tunnel: [w621 1 0 w626] -> w619
              tunnel: [w621 0 1 w626] -> w618
              frame .."Lin - Lin" {
                w621 = 0
              }
              frame "Log - Lin" {
              }
              frame "Lin - Log" {
              }
              frame "Log - log".. {
                w626 = 1
              }
            }
            n323 = property on="Cgraph" class="WFGraph (strict)"("X Scale.Mapping Mode"=w619) -> ()  [unwired: 2 in, 2 out]
            n324 = property on="Cgraph" class="WFGraph (strict)"("Y Scale.Mapping Mode"=w618, "YScale.Minimum"=w618) -> ()  [unwired: 2 in, 2 out]
          }
        }
        n325 = case shown="True" w585 {
          tunnel: w590 -> [_ w598]
          frame False {
          }
          frame True {
            n326 = property on="Cgraph" class="WFGraph (strict)"() -> ("YScale.Mapping Mode"=w601:u8)  [unwired: 2 in, 2 out]
            n327 = global read "QC_MeasurementSetup.vi" "CV Measurement Parameters"() -> (w600:T8)
            n328 = property on="Cgraph" class="WFGraph (strict)"("YScale.Minimum"=w601) -> ()  [unwired: 2 in, 2 out]
            n329 = Unbundle By Name(w600) -> ("Initial Voltage [V]"=w603:dbl, "Step Size [V]"=w605:dbl, "Number Of Steps"=w602:u32)
            n330 = call "CVData.vi"("Action"=T3."Read Array", "Array No."=u32 1 ("Action")) -> ("Array OUT"=w594:dbl[])  [unwired: 3 in, 1 out]
            n331 = Absolute Value(x=w605) -> (abs(x)=w604:dbl)
            n332 = Array Subset(array=w594, index=0, length=w602) -> (w606:dbl[])
            n333 = Absolute Value(x=w606) -> (abs(x)=w599:dbl[])
            n334 = case shown="..\"1/C^2 [1/nF^2]\"" w598 {
              tunnel: [w611 w614 w617] -> w597
              tunnel: w599 -> [w609 w616 w617]
              frame .."1/C^2 [1/nF^2]" {
                n335 = Array Size(array=w609) -> (size(s)=w610:i32)
                n336 = for {
                  N: w610 -> [_]
                  tunnel: w609 -> [w613] mode=indexing
                  tunnel: [w612] -> w611 mode=indexing
                  n337 = formula code="y=1000000./(x*x);"("x"=w613) -> ("y"=w612:dbl)
                }
              }
              frame "nF" {
                n338 = Divide(x=w616, y=1000.0) -> (x/y=w614:dbl[])
              }
              frame "pF".. {
              }
            }
            n339 = Bundle("Initial Voltage [V]"=w603, w604, w597) -> (w607:cluster{"Initial Voltage [V]":dbl, dbl, dbl[]})  [unwired: 1 in]
            n340 = local write "Cgraph"(w607) -> ()
          }
        }
        n341 = Not Or(1:"quit (no save)", 2:"Quit & Save") -> (0:w588:bool)
      }
      n342 = global read "QC_MeasurementSetup.vi" "CV Measurement Parameters"() -> (w539:T8)
      n343 = Unbundle By Name(w539) -> ("Temperature Readout"=w538:enum16{"Read Arduino", "Enter manually"}, "Arduino"=w532:refnum<class "ArduinoControl.lvclass">)
      n344 = case shown="\"Read Arduino\"" w538 {
        tunnel: w532 -> [_ w584]
        frame "Enter manually", Default {
        }
        frame "Read Arduino" {
          n345 = call "ArduinoClose.vi"("ArduinoControl in"=w584) -> ()  [unwired: 9 in, 2 out]
        }
      }
      n346 = case shown="True" w542 {
        tunnel: [FALSE w628] -> w544
        frame False {
        }
        frame True {
          n347 = Two Button Dialog(message="Are you sure you don't want to save the data?", 1:"Quit" ("F button name (\"Cancel\")"), 2:"Save data" ("T button name (\"OK\")")) -> (T button?=w628:bool)
        }
      }
      n348 = Or(x=w543, y=w544) -> (x .or. y?=w537:bool)
      n349 = flat-sequence {
        tunnel: w537 -> [w546]
        tunnel: [w546] -> w533
        tunnel: [TRUE] -> w531
        frame #0 {
          n350 = global read "QC_MeasurementSetup.vi" "CV Measurement Parameters"() -> (w556:T8)
          n351 = Unbundle By Name(w556) -> ("V_depletion Limit [V]"=w548:dbl, "Number Of Steps"=w551:u32)
          n352 = call "ScanFeedback.vi"("measurement type"=T5."CV") -> ("V depletion"=w550:dbl)  [unwired: 4 in, 4 out]
          n353 = case shown="True" w546 {
            tunnel: ["" w583] -> w557
            tunnel: [_ w566] -> w555
            tunnel: w551 -> [_ w563]
            frame False {
            }
            frame True {
              w564 = T3."Read Array" ("Action")
              n354 = local write "STATUS 1"("Saving Data ...") -> ()
              n355 = call "CVData.vi"("Action"=w564, "Array No."=u32 2 ("Action")) -> ("Array OUT"=w561:dbl[])  [unwired: 3 in, 1 out]
              n356 = Multiply(x=w561, y=0.001) -> (x*y=w560:dbl[])
              n357 = call "CVData.vi"("Action"=w564, "Array No."=u32 0 ("Action")) -> ("Array OUT"=w573:dbl[])  [unwired: 3 in, 1 out]
              n358 = call "CVData.vi"("Action"=w564, "Array No."=u32 1 ("Action")) -> ("Array OUT"=w572:dbl[])  [unwired: 3 in, 1 out]
              n359 = Build Array(w573, w572, w560) -> (w571:dbl[][])
              n360 = call "CVData.vi"("Action"=w564, "Array No."=u32 4 ("Action")) -> ("Array OUT"=w579:dbl[])  [unwired: 3 in, 1 out]
              n361 = call "CVData.vi"("Action"=w564, "Array No."=u32 3 ("Action")) -> ("Array OUT"=w578:dbl[])  [unwired: 3 in, 1 out]
              n362 = call <vilib>:"Std Deviation and Variance.vi"("X"=w579) -> ("mean"=w567:dbl)  [unwired: 1 in, 2 out]
              n363 = call <vilib>:"Std Deviation and Variance.vi"("X"=w578) -> ("mean"=w568:dbl)  [unwired: 1 in, 2 out]
              n364 = Transpose 2D Array(2D array=w571) -> (transposed array=w570:dbl[][])
              n365 = call "SaveDataFile.vi"("Data Array"=w570, "Temperature"=w568, "Humidity"=w567, "no. of arrays"=3, "Actual array lengths"=w563, "Array Titles"="Voltage[V] Capacitance[pF] Resistance[kOhm]", "Strip Segment"="", "Arrays format"="%010.2f") -> ("Path + Filename OUT"=w583:string, "Error Out"=w566:errorcluster)  [unwired: 4 in, 2 out]
            }
          }
          n366 = Absolute Value(x=w550) -> (abs(x)=w549:dbl)
          n367 = Absolute Value(x=w548) -> (abs(x)=w547:dbl)
          n368 = Less Or Equal?(x=w549, y=w547) -> (x <= y?=w552:bool)
          n369 = call "WriteLogFile.vi"("Automatic warning"="", "Data File"=w557, "Error In"=w555, "DUT passed?"=w552, "Value TechSpec criteria"=w550, "Files saved?"=w546) -> ()  [unwired: 5 in, 1 out]
        }
      }
      n370 = Select(t="Run finished.\nData saved." ("STATUS 1"), s=w533, f="Run finished.\nData not saved." ("STATUS 1")) -> (s? t:f=w536:string)
      n371 = local write "STATUS 1"(w536) -> ()
      "Done!" <- w531
    }
  }
